vi "check arduino parse error (sub-vi).vi"(11 "error":errorcluster) -> (2 "is arduino parse error?":bool)   [LabVIEW 2021]
uses:
  type-defs/project_custom_error_codes_ring (type def).ctl
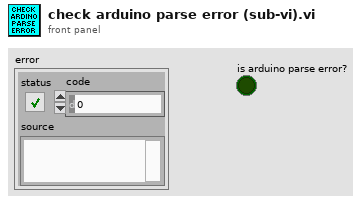
[diagram p1: front panel]
types:
  T1 = typedef "project_custom_error_codes_ring (type def).ctl" = i32
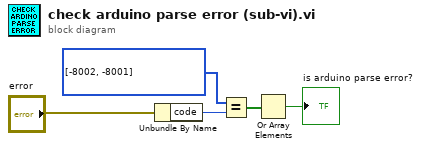
[diagram p0: block diagram]
diagram:
  w4 = T1[] [-8002, -8001] items=["parse_failure"=-8001, "arduino_failure"=-8002] ("Array")
  n1 = Unbundle By Name("error") -> ("code"=w5:i32)
  n2 = Equal?(x=w4, y=w5) -> (x = y?=w3:bool[])
  n3 = Or Array Elements(Boolean array=w3) -> (logical OR=→"is arduino parse error?":bool)
